vi "Set MeasData in Q.vi"(6 "UpdateTS (T)":bool=TRUE, 8 "error in (no error)":errorcluster, 10 "MeasData out":T1) -> (0 "error out":errorcluster, 3 "orData out":T3)   [LabVIEW 2019]
doc: "Developed by Kevin Thompson\nThompson Engineering, LLC\nkevin@thompsonengineering.net"
uses:
  TD MeasData QRef.ctl
  TD MeasData--cluster.ctl
  DataTypes/InverterPhaseData--cluster.ctl
  GBL DataQ Ref.vi
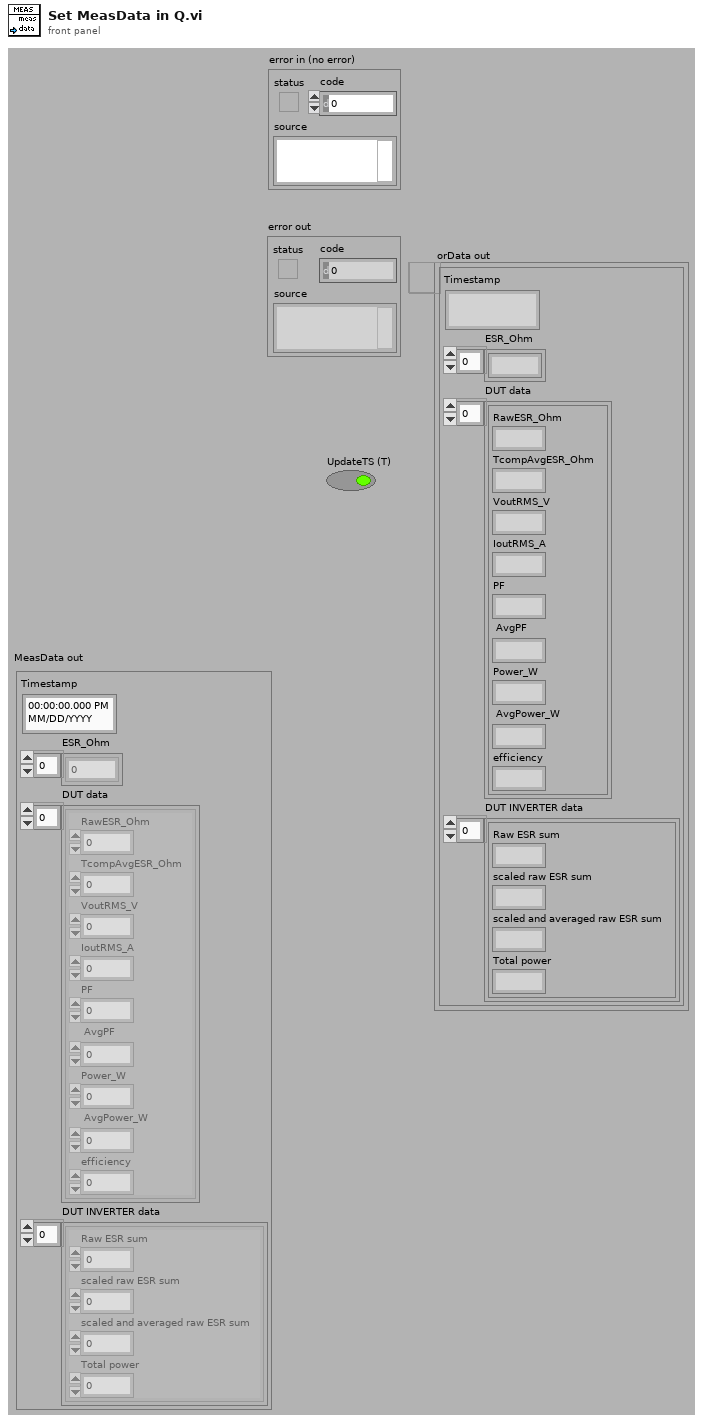
[diagram p1: front panel]
types:
  T1 = typedef "TD MeasData--cluster.ctl" = cluster{"Timestamp":timestamp, "ESR_Ohm":dbl[], "DUT data":T2[], "DUT INVERTER data":cluster{"Raw ESR sum":dbl, "scaled raw ESR sum":dbl, "scaled and averaged raw ESR sum":dbl, "Total power":dbl}[]}
  T2 = typedef "InverterPhaseData--cluster.ctl" = cluster{"RawESR_Ohm":dbl, "TcompAvgESR_Ohm":dbl, "VoutRMS_V":dbl, "IoutRMS_A":dbl, "PF":dbl, "AvgPF":dbl, "Power_W":dbl, "AvgPower_W":dbl, "efficiency":dbl}
  T3 = typedef "TD MeasData QRef.ctl" = refnum<queue>
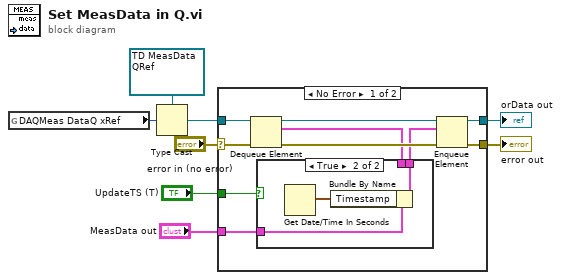
[diagram p0: block diagram]
diagram:
  n1 = global read "GBL DataQ Ref.vi" "DAQMeas DataQ xRef"() -> (w3:u32)
  n2 = Type Cast(type=T3 refnum ("orData in"), x=w3) -> (*(type *) &x=w4:T3)
  n3 = case shown="No Error" "error in (no error)" {
    selector: "error in (no error)" -> [w13 w23]
    tunnel: w4 -> [w18 w24]
    tunnel: [w15 w23] -> w8
    tunnel: [w14 w24] -> w7
    tunnel: "MeasData out" -> [w10 _]
    tunnel: "UpdateTS (T)" -> [w9 _]
    frame No Error {
      n4 = Dequeue Element(queue=w18, error in (no error)=w13) -> (queue out=w16:T3, element=w12:T1, error out=w17:errorcluster)  [unwired: 1 in, 1 out]
      n5 = case shown="True" w9 {
        tunnel: w12 -> [_ _]
        tunnel: [w19 w21] -> w11
        tunnel: w10 -> [w19 w22]
        frame False {
        }
        frame True {
          n6 = Get Date/Time In Seconds() -> (seconds since 1Jan1904=w20:timestamp)
          n7 = Bundle By Name(cluster=w22, "Timestamp"=w20) -> (w21:T1)
        }
      }
      n8 = Enqueue Element(queue=w16, element=w11, error in (no error)=w17) -> (queue out=w14:T3, error out=w15:errorcluster)  [unwired: 1 in, 1 out]
    }
    frame Error {
    }
  }
  "orData out" <- w7
  "error out" <- w8
